vi "Get Application Name.vi"() -> (3 "Application Name":string)   [LabVIEW 2020]
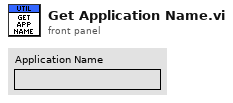
[diagram p1: front panel]
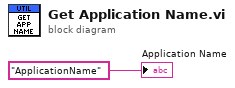
[diagram p0: block diagram]
diagram:
  "Application Name" <- "ApplicationName" ("Application Name")
